vi "worksheet filter list.vi"(8 "error in (no error)":errorcluster, 9 "list":string[](array[string]), 10 "col":u16, 11 "worksheet":u32) -> (0 "error out":errorcluster, 3 "function return":u32(ring))   [LabVIEW 8.6]
doc: "lxw_error worksheet_filter_list(lxw_worksheet worksheet, lxw_col_t col, unsigned long list);"
uses:
  pending_lvxlsxwriter/xlsxwriter.dll
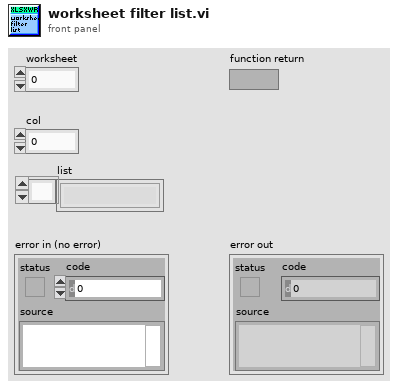
[diagram p1: front panel]
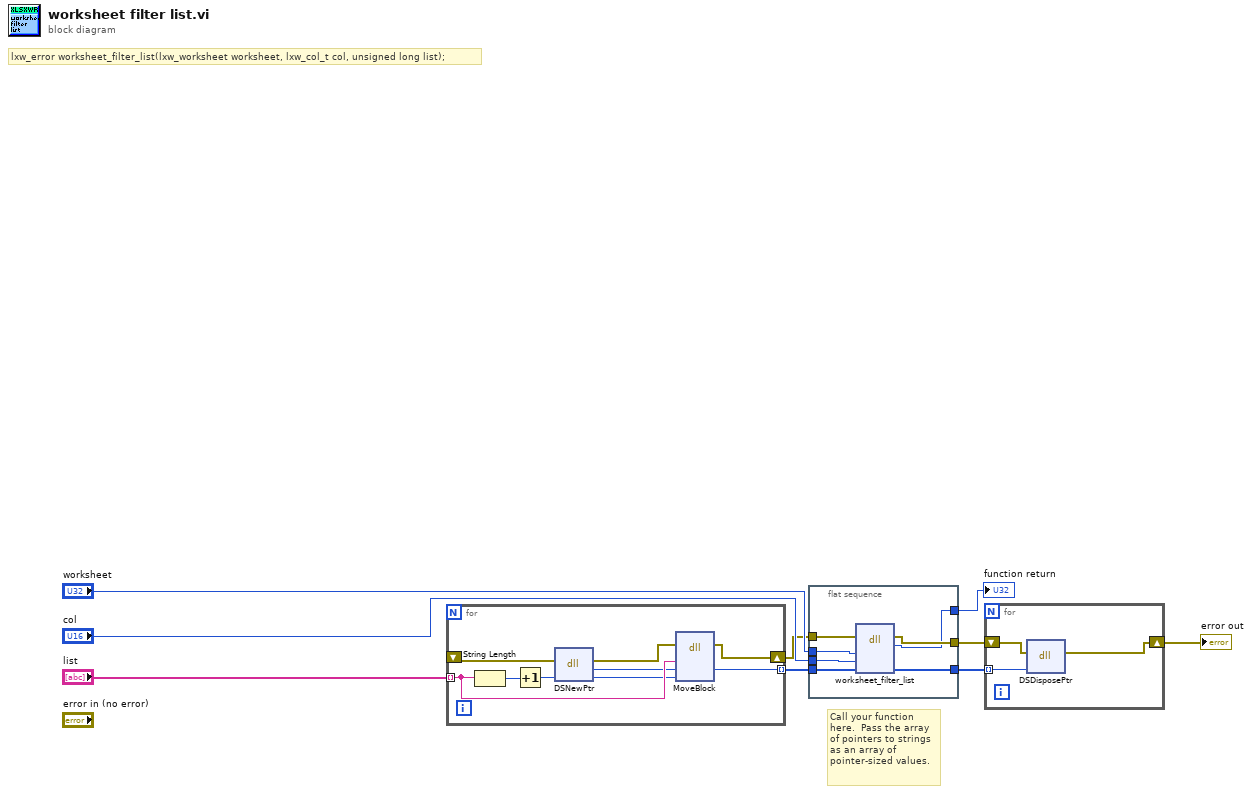
[diagram p0: block diagram]
diagram:
  # "Call your function\nhere.  Pass the array\nof pointers to strings\nas an array of\npointer-sized values."
  # "lxw_error worksheet_filter_list(lxw_worksheet worksheet, lxw_col_t col, unsigned long list);"
  n1 = for {
    tunnel: "list" -> [w16] mode=indexing
    tunnel: [w12] -> w9 mode=indexing
    shift-right: [w10] -> w4
    shift-left: _ -> [w11]
    n2 = String Length(string=w16) -> (length=w18:i32)
    n3 = Increment(x=w18) -> (x+1=w17:i32)
    n4 = dll-call lib="LabVIEW" fn="DSNewPtr"(error in=w11, "size"=w17) -> (error out=w13:errorcluster, "return type"=w15:u64, "size"=w14:u32)  [unwired: 2 in, 1 out]
    n5 = dll-call lib="LabVIEW" fn="MoveBlock"(error in=w13, "pSrc"=w16, "pDst"=w15, "size"=w14) -> (error out=w10:errorcluster, "pDst"=w12:u64)  [unwired: 5 in, 1 out]
  }
  n6 = flat-sequence {
    tunnel: w9 -> [w25]
    tunnel: [w24] -> w8
    tunnel: "col" -> [w23]
    tunnel: "worksheet" -> [w22]
    tunnel: w4 -> [w21]
    tunnel: [w20] -> w3
    tunnel: [w19] -> w2
    frame #0 {
      n7 = dll-call lib="C:/Users/WDAGUtilityAccount/Desktop/pending_lvxlsxwriter/xlsxwriter.*" fn="worksheet_filter_list"(error in=w21, "worksheet"=w22, "col"=w23, "list"=w25) -> (error out=w20:errorcluster, "return type"=w19:u32, "list"=w24:u64[])  [unwired: 4 in, 1 out]
    }
  }
  n8 = for {
    tunnel: w8 -> [w28] mode=indexing
    shift-right: [w26] -> w1
    shift-left: w3 -> [w27]
    n9 = dll-call lib="LabVIEW" fn="DSDisposePtr"(error in=w27, "ptr"=w28) -> (error out=w26:errorcluster)  [unwired: 4 in, 1 out]
  }
  "error out" <- w1
  "function return" <- w2
